vi "Checks_Relative Offset Uniqueness.vi"(8 "error in (no error)":errorcluster, 11 "DMA":T1) -> (0 "error out":errorcluster)   [LabVIEW 2017, in "GE_RM_System Explorer.lvlib"]
doc: "This VI checks that, for a given DMA Block, all Channels Relative Offset are unique."
uses:
  GE_RM_System Explorer.lvlib
  Typedef_DMA Instance.ctl
  Typedef_DMA Block Settings.ctl
  Shared/Data Channel Type.ctl
  Typedef_Channel Settings.ctl
  <userlib>/_OpenG.lib/array/array.llb/Remove Duplicates from 1D Array (U32)__ogtk.vi
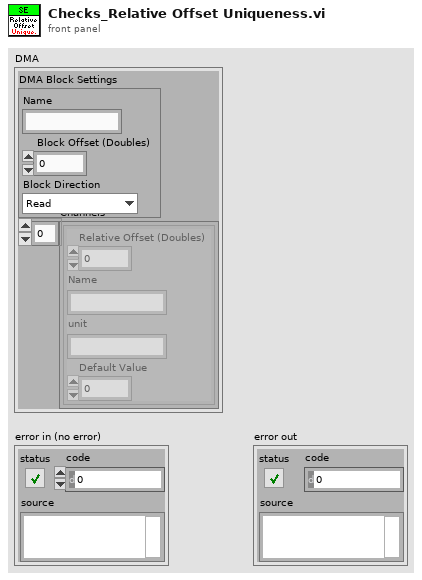
[diagram p1: front panel]
types:
  T1 = typedef "GE_RM_System Explorer.lvlib/Typedef_DMA Instance.ctl" = cluster{"DMA Block Settings":T2, "Channels":T4[]}
  T2 = typedef "GE_RM_System Explorer.lvlib/Typedef_DMA Block Settings.ctl" = cluster{"Name":string, " Block Offset (Doubles)":u32, "Block Direction":T3}
  T3 = typedef "GE_RM_System Explorer.lvlib/Data Channel Type.ctl" = enum16{"Read", "Write"}
  T4 = typedef "GE_RM_System Explorer.lvlib/Typedef_Channel Settings.ctl" = cluster{"Relative Offset (Doubles)":u32, "Name":string, "unit":string, "Default Value":dbl}
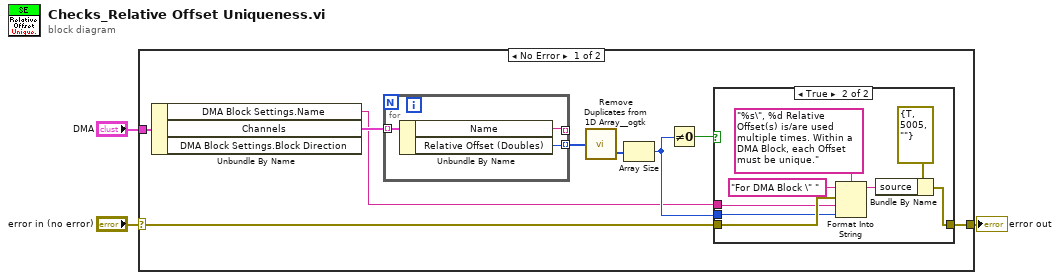
[diagram p0: block diagram]
diagram:
  n1 = case shown="No Error" "error in (no error)" {
    selector: "error in (no error)" -> [w8 w25]
    tunnel: [w7 w25] -> w3
    tunnel: "DMA" -> [w10 _]
    frame No Error {
      n2 = Unbundle By Name(w10) -> ("DMA Block Settings.Name"=w4:string, "Channels"=w11:T4[])  [unwired: 1 out]
      n3 = for {
        tunnel: w11 -> [w23] mode=indexing
        tunnel: [w24] -> _ mode=indexing
        tunnel: [w22] -> w12 mode=indexing
        n4 = Unbundle By Name(w23) -> ("Name"=w24:string, "Relative Offset (Doubles)"=w22:u32)
      }
      n5 = call-poly <userlib>:"Remove Duplicates from 1D Array__ogtk.vi"("Input Array"=w12) -> ("indices of removed elements"=w6:i32[])  [unwired: 1 out]
      n6 = Array Size(array=w6) -> (size(s)=w5:i32)
      n7 = Not Equal To 0?(x=w5) -> (x != 0?=w9:bool)
      n8 = case shown="True" w9 {
        tunnel: w8 -> [w13 w18]
        tunnel: [w13 w19] -> w7
        tunnel: w5 -> [_ w17]
        tunnel: w4 -> [_ w14]
        frame False {
        }
        frame True {
          n9 = Format Into String(format string="%s\", %d Relative Offset(s) is/are used multiple times. Within a DMA Block, each Offset must be unique.", initial string="For DMA Block \" ", error in=w18, w14, w17) -> (resulting string=w20:string)  [unwired: 1 out]
          n10 = Bundle By Name(cluster=errorcluster {"status"=TRUE, "code"=5005, "source"=""} ("error IO"), "source"=w20) -> (w19:errorcluster)
        }
      }
    }
    frame Error {
    }
  }
  "error out" <- w3
